vi "updateGUIClosedLoopParams.vi"(11 "Data Cluster in":T1) -> (3 "Data Cluster out":T1)   [LabVIEW 2015]
uses:
  controls/UI Data.ctl
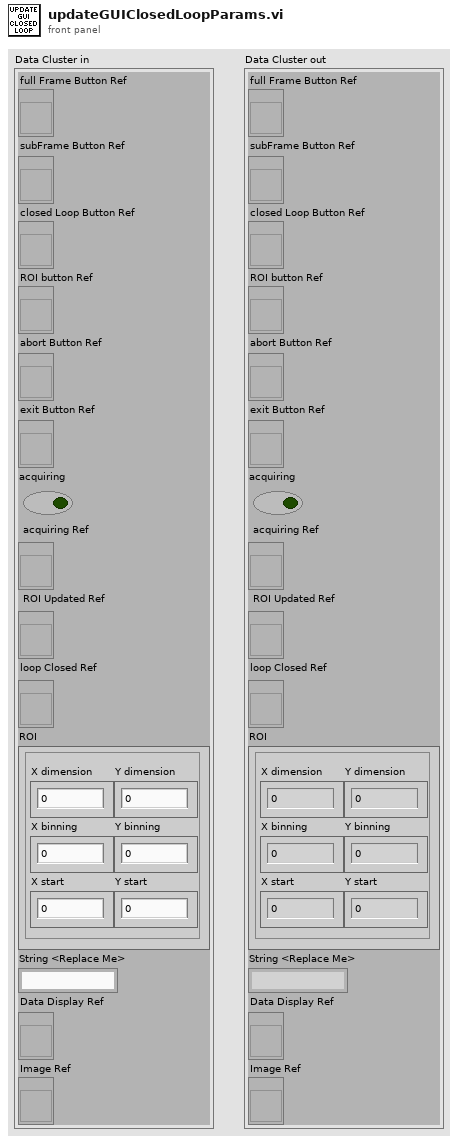
[diagram p1: front panel]
types:
  T1 = typedef "UI Data.ctl" = cluster{"full Frame Button Ref":refnum<vi>, "subFrame Button Ref":refnum<vi>, "closed Loop Button Ref":refnum<vi>, "ROI button Ref":refnum<vi>, "abort Button Ref":refnum<vi>, "exit Button Ref":refnum<vi>, "acquiring":bool, " acquiring Ref":refnum<vi>, " ROI Updated Ref":refnum<vi>, "loop Closed Ref":refnum<vi>, "ROI":cluster{"X dimension":i16, "Y dimension":i16, "X binning":i16, "Y binning":i16, "X start":i16, "Y start":i16}, "String <Replace Me>":string, "Data Display Ref":refnum<vi>, "Image Ref":refnum<vi>}
  T2 = enum8{"Enabled", "Disabled", "Disabled and Grayed Out"}
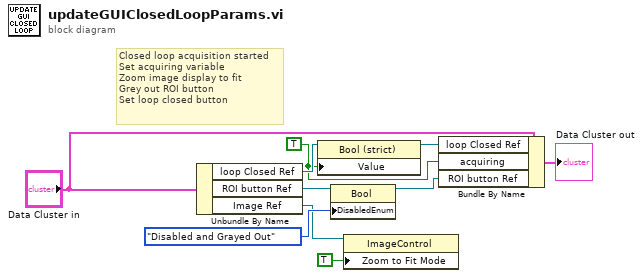
[diagram p0: block diagram]
diagram:
  w2 = TRUE ("acquiring")
  # "Closed loop acquisition started\nSet acquiring variable\nZoom image display to fit\nGrey out ROI button\nSet loop closed button"
  n1 = Unbundle By Name("Data Cluster in") -> ("loop Closed Ref"=w3:refnum<vi>, "ROI button Ref"=w8:refnum<vi>, "Image Ref"=w6:refnum<vi>)
  n2 = property class="Bool (strict)"(reference=w3, "Value"=w2) -> (reference out=w1:refnum<vi>)  [unwired: 1 in, 1 out]
  n3 = property class="Bool"(reference=w8, "DisabledEnum"=T2."Disabled and Grayed Out" ("Disabled")) -> (reference out=w10:refnum<vi>)  [unwired: 1 in, 1 out]
  n4 = property class="ImageControl"(reference=w6, "Zoom to Fit Mode"=TRUE) -> ()  [unwired: 1 in, 2 out]
  n5 = Bundle By Name(cluster="Data Cluster in", "loop Closed Ref"=w1, "acquiring"=w2, "ROI button Ref"=w10) -> (→"Data Cluster out":T1)
